vi "Inquiring_and_setting_parameters_Reglo_D.vi"(5 "Parameter":string, 7 "Command":T1=enum."Pump type/Software version/Pump head ?", 8 "error in (no error)":errorcluster, 11 "Pumpe":T2=enum."P_01") -> (0 "error out":errorcluster, 3 "Answer":string)   [LabVIEW 2019]
doc: "Sended den gewünschten Befehl an die selektierte Pumpe.\n\nSends the elected order to the defined pumpl.\n\nÜbernommen von Zühlke/AV\n\n24.11.2003 - Ismatec/CS"
uses:
  Pumpen.ctl
  Inquiring_and_setting_parameters_Reglo_D.ctl
panel:
  in  "VISA resource name In":refnum<visa-resource-name>="COM1"
  out "Parameter wrong":bool
  # "Wrong length or\nwrong value"
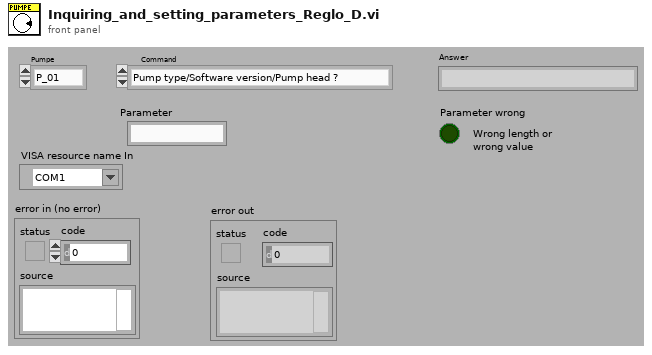
[diagram p1: front panel]
types:
  T1 = typedef "Inquiring_and_setting_parameters_Reglo_D.ctl" = enum16{"Current Mode active/inactive ?", "Pump type/Software version/Pump head ?", "Software version ?", "Speed ?", "Speed !", "Default flow rate ?", "Calibrated flow rate ?", "Calibrated flow rate !", "Number of digits after dec.point ?", "Pump tubing inner diameter ?", "Pump tubing inner diameter !", "Dispensing time in 1/10 sec. ?", "Dispensing time in 1/10 sec. !", "Dispensing time in minutes !", "Dispensing time in hours !", "Roller steps for \"MODE DISP - Volume\" ?", "Roller steps for \"MODE DISP - Volume\" !", "Dispensing volume in ml for \"MODE DISP - Volume\" !", "Roller back steps ?", "Roller back steps !", "Pause time in 1/10 sec ?", "Pause time in 1/10 sec. !", "Pause time in minutes !", "Pause time in hours !", "Number of dispensing cycles ?", "Number of dispensing cycles !", "Delivered titration volume ?", "Reset titration volume to 0", "Store application parameters", "Set default values", "Foot switch ?"}
  T2 = typedef "Pumpen.ctl" = enum16{"Pumpe mit Adresse 0 gibt es nicht", "P_01", "P_02", "P_03", "P_04", "P_05", "P_06", "P_07", "P_08"}
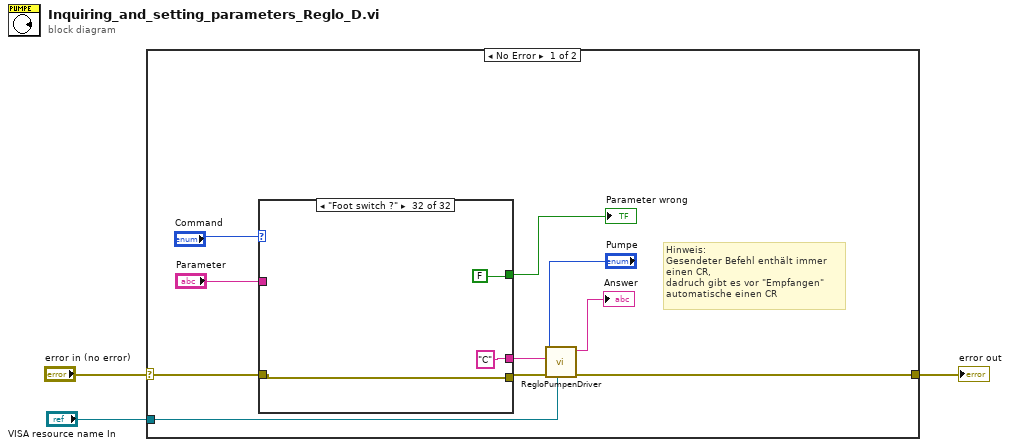
[diagram p0: block diagram]
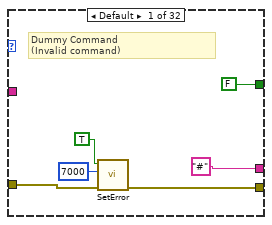
[diagram p2: hidden frame]
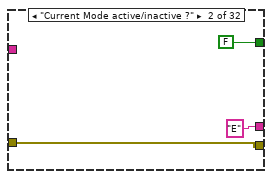
[diagram p3: hidden frame]
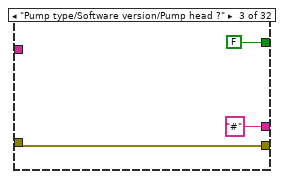
[diagram p4: hidden frame]
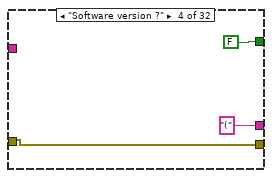
[diagram p5: hidden frame]
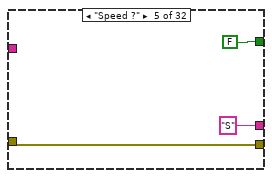
[diagram p6: hidden frame]
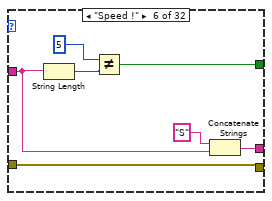
[diagram p7: hidden frame]
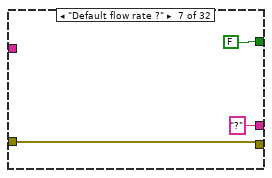
[diagram p8: hidden frame]
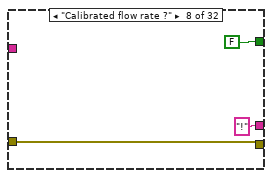
[diagram p9: hidden frame]
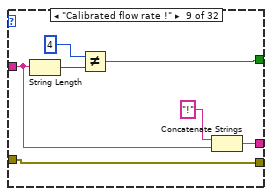
[diagram p10: hidden frame]
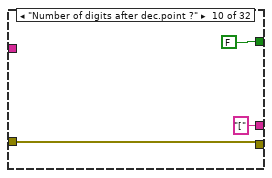
[diagram p11: hidden frame]
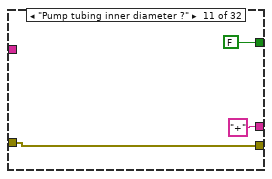
[diagram p12: hidden frame]
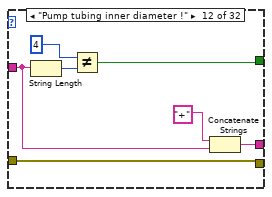
[diagram p13: hidden frame]
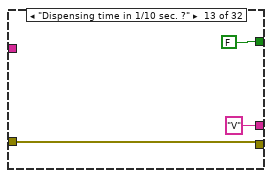
[diagram p14: hidden frame]
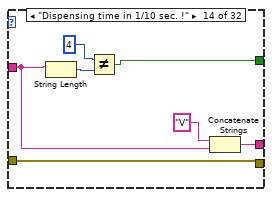
[diagram p15: hidden frame]
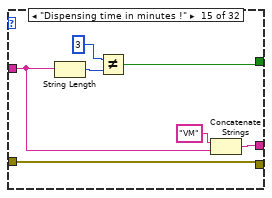
[diagram p16: hidden frame]
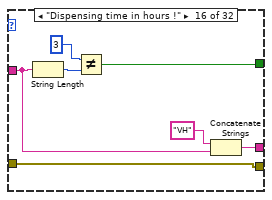
[diagram p17: hidden frame]
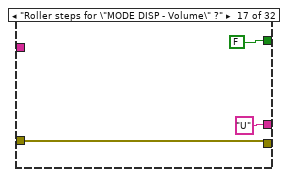
[diagram p18: hidden frame]
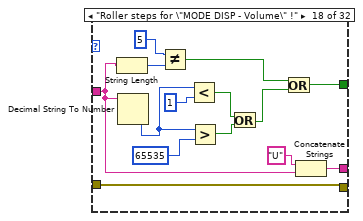
[diagram p19: hidden frame]
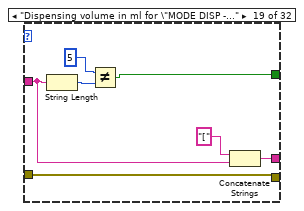
[diagram p20: hidden frame]
diagram:
  n1 = case shown="No Error" "error in (no error)" {
    selector: "error in (no error)" -> [w12 w179]
    tunnel: [w7 w179] -> w2
    tunnel: "VISA resource name In" -> [w4 _]
    frame No Error {
      # "Hinweis:\nGesendeter Befehl enthält immer einen CR,\ndadruch gibt es vor \"Empfangen\"  automatische einen CR"
      n2 = case shown="\"Foot switch ?\"" "Command" {
        tunnel: [w19 w22 w24 w27 w30 w38 w40 w43 w45 w52 w56 w58 w65 w68 w75 w84 w91 w105 w110 w115 w129 w131 w134 w144 w150 w154 w158 w166 w169 w171 w175 w177] -> w11
        tunnel: w12 -> [w18 w22 w24 w27 w30 w38 w40 w43 w45 w52 w56 w58 w65 w68 w75 w84 w91 w105 w110 w115 w129 w131 w134 w144 w150 w154 w158 w166 w169 w171 w175 w177]
        tunnel: ["#" ("Parameter") "E" ("Parameter") "#" ("Parameter") "(" ("Parameter") "S" ("Parameter") w37 "?" ("Parameter") "!" ("Parameter") w51 "[" ("Parameter") "+" ("Parameter") w64 "V" ("Parameter") w71 w78 w86 "U" ("Parameter") w102 w108 "%" ("Parameter") w128 "T" ("Parameter") w136 w143 w149 "\"" ("Parameter") w160 ":" ("Parameter") "W" ("Parameter") "*" ("Parameter") "0" ("Parameter") "C" ("Parameter")] -> w9
        tunnel: "Parameter" -> [_ _ _ _ _ w36 _ _ w46 _ _ w62 _ w70 w77 w85 _ w101 w107 _ w116 _ w135 w142 w148 _ w159 _ _ _ _ _]
        tunnel: [FALSE FALSE FALSE FALSE FALSE w32 FALSE FALSE w47 FALSE FALSE w59 FALSE w72 w79 w82 FALSE w93 w109 FALSE w118 FALSE w137 w140 w151 FALSE w161 FALSE FALSE FALSE FALSE FALSE] -> w6
        frame Default {
          # "Dummy Command\n(Invalid command)"
          n3 = call "SetError.vi"("error in"=w18, "error code"=7000, "Error?"=TRUE) -> ("error out"=w19:errorcluster)  [unwired: 6 in]
        }
        frame "Current Mode active/inactive ?" {
        }
        frame "Pump type/Software version/Pump head ?" {
        }
        frame "Software version ?" {
        }
        frame "Speed ?" {
        }
        frame "Speed !" {
          n4 = String Length(string=w36) -> (length=w34:i32)
          n5 = Not Equal?(x=5 ("y"), y=w34) -> (x != y?=w32:bool)
          n6 = Concatenate Strings("S" ("Parameter"), w36) -> (w37:string)
        }
        frame "Default flow rate ?" {
        }
        frame "Calibrated flow rate ?" {
        }
        frame "Calibrated flow rate !" {
          n7 = String Length(string=w46) -> (length=w49:i32)
          n8 = Not Equal?(x=4, y=w49) -> (x != y?=w47:bool)
          n9 = Concatenate Strings("!" ("Parameter"), w46) -> (w51:string)
        }
        frame "Number of digits after dec.point ?" {
        }
        frame "Pump tubing inner diameter ?" {
        }
        frame "Pump tubing inner diameter !" {
          n10 = String Length(string=w62) -> (length=w61:i32)
          n11 = Not Equal?(x=4, y=w61) -> (x != y?=w59:bool)
          n12 = Concatenate Strings("+" ("Parameter"), w62) -> (w64:string)
        }
        frame "Dispensing time in 1/10 sec. ?" {
        }
        frame "Dispensing time in 1/10 sec. !" {
          n13 = String Length(string=w70) -> (length=w74:i32)
          n14 = Not Equal?(x=4, y=w74) -> (x != y?=w72:bool)
          n15 = Concatenate Strings("V" ("Parameter"), w70) -> (w71:string)
        }
        frame "Dispensing time in minutes !" {
          n16 = String Length(string=w77) -> (length=w81:i32)
          n17 = Not Equal?(x=3, y=w81) -> (x != y?=w79:bool)
          n18 = Concatenate Strings("VM" ("Parameter"), w77) -> (w78:string)
        }
        frame "Dispensing time in hours !" {
          n19 = String Length(string=w85) -> (length=w88:i32)
          n20 = Not Equal?(x=3, y=w88) -> (x != y?=w82:bool)
          n21 = Concatenate Strings("VH" ("Parameter"), w85) -> (w86:string)
        }
        frame "Roller steps for \"MODE DISP - Volume\" ?" {
        }
        frame "Roller steps for \"MODE DISP - Volume\" !" {
          n22 = String Length(string=w101) -> (length=w104:i32)
          n23 = Decimal String To Number(string=w101) -> (number=w100:i32)  [unwired: 2 in, 1 out]
          n24 = Not Equal?(x=5, y=w104) -> (x != y?=w97:bool)
          n25 = Less?(x=w100, y=1) -> (x < y?=w95:bool)
          n26 = Greater?(x=w100, y=65535) -> (0:w94:bool)
          n27 = Or(x=w95, y=w94) -> (x .or. y?=w96:bool)
          n28 = Or(x=w97, y=w96) -> (x .or. y?=w93:bool)
          n29 = Concatenate Strings("U" ("Parameter"), w101) -> (w102:string)
        }
        frame "Dispensing volume in ml for \"MODE DISP - Volume\" !" {
          n30 = String Length(string=w107) -> (length=w112:i32)
          n31 = Not Equal?(x=5, y=w112) -> (x != y?=w109:bool)
          n32 = Concatenate Strings("[" ("Parameter"), w107) -> (w108:string)
        }
        frame "Roller back steps ?" {
        }
        frame "Roller back steps !" {
          n33 = String Length(string=w116) -> (length=w126:i32)
          n34 = Decimal String To Number(string=w116) -> (number=w124:i32)  [unwired: 2 in, 1 out]
          n35 = Not Equal?(x=4, y=w126) -> (x != y?=w122:bool)
          n36 = Less?(x=w124, y=0) -> (x < y?=w120:bool)
          n37 = Greater?(x=w124, y=100) -> (0:w119:bool)
          n38 = Or(x=w120, y=w119) -> (x .or. y?=w121:bool)
          n39 = Or(x=w122, y=w121) -> (x .or. y?=w118:bool)
          n40 = Concatenate Strings("%" ("Parameter"), w116) -> (w128:string)
        }
        frame "Pause time in 1/10 sec ?" {
        }
        frame "Pause time in 1/10 sec. !" {
          n41 = String Length(string=w135) -> (length=w139:i32)
          n42 = Not Equal?(x=4, y=w139) -> (x != y?=w137:bool)
          n43 = Concatenate Strings("T" ("Parameter"), w135) -> (w136:string)
        }
        frame "Pause time in minutes !" {
          n44 = String Length(string=w142) -> (length=w146:i32)
          n45 = Not Equal?(x=3, y=w146) -> (x != y?=w140:bool)
          n46 = Concatenate Strings("TM" ("Parameter"), w142) -> (w143:string)
        }
        frame "Pause time in hours !" {
          n47 = String Length(string=w148) -> (length=w153:i32)
          n48 = Not Equal?(x=3, y=w153) -> (x != y?=w151:bool)
          n49 = Concatenate Strings("TH" ("Parameter"), w148) -> (w149:string)
        }
        frame "Number of dispensing cycles ?" {
        }
        frame "Number of dispensing cycles !" {
          n50 = String Length(string=w159) -> (length=w163:i32)
          n51 = Not Equal?(x=4, y=w163) -> (x != y?=w161:bool)
          n52 = Concatenate Strings("\"" ("Parameter"), w159) -> (w160:string)
        }
        frame "Delivered titration volume ?" {
        }
        frame "Reset titration volume to 0" {
        }
        frame "Store application parameters" {
        }
        frame "Set default values" {
        }
        frame "Foot switch ?" {
        }
      }
      "Parameter wrong" <- w6
      n53 = call "RegloPumpenDriver.vi"("VISA resource name In"=w4, "error in"=w11, "Befehl"=w9, "Pump"="Pumpe") -> ("error out"=w7:errorcluster, "Receivestring"=→"Answer":string)  [unwired: 3 in, 3 out]
    }
    frame Error {
    }
  }
  "error out" <- w2
